vi "calc_min_vswr.vi"(11 "plot_log_phase_vswr":cluster{"freq_array_out":dbl[], dbl[]}[](array[cluster])) -> (0 "min_vswr_idx":i32, 2 "min_vswr":dbl, 3 "min_vswr_freq":string)   [LabVIEW 2025]
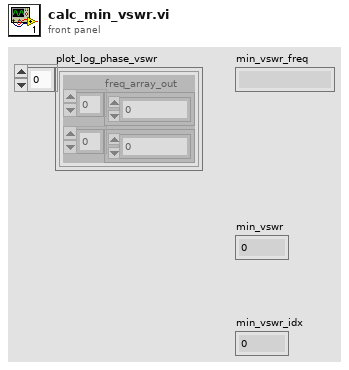
[diagram p1: front panel]
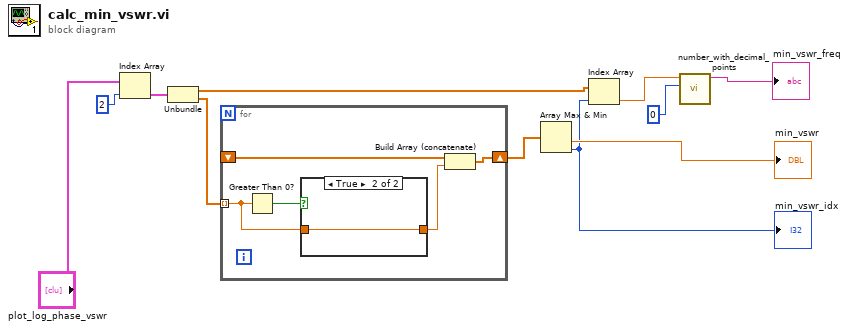
[diagram p0: block diagram]
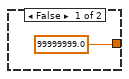
[diagram p2: hidden frame]
diagram:
  n1 = Index Array(array="plot_log_phase_vswr", index=2) -> (element=w8:cluster{"freq_array_out":dbl[], dbl[]})
  n2 = Unbundle(w8) -> ("freq_array_out"=w4:dbl[], w2:dbl[])
  n3 = for {
    tunnel: w2 -> [w14] mode=indexing
    shift-right: [w13] -> w1
    shift-left: _ -> [w12]
    n4 = Greater Than 0?(x=w14) -> (x > 0?=w16:bool)
    n5 = case shown="True" w16 {
      tunnel: [99999999.0 ("phase") w18] -> w15
      tunnel: w14 -> [_ w18]
      frame False {
      }
      frame True {
      }
    }
    n6 = Build Array (concatenate)(w12, w15) -> (w13:dbl[])
  }
  n7 = Array Max & Min(array=w1) -> (min value=→"min_vswr":dbl, min index (indices)=w7:i32)  [unwired: 2 out]
  "min_vswr_idx" <- w7
  n8 = Index Array(array=w4, index=w7) -> (element=w5:dbl)
  n9 = call "number_with_decimal_points.vi"("Precision"=i16 0, "Double"=w5) -> ("String"=→"min_vswr_freq":string)  [unwired: 5 in]
